vi "stop.vi"(8 "error in (no error)":errorcluster, 9 "InternalCommandId.lvclass":refnum<class "InternalCommandId.lvclass">, 10 "ElectrometerController in":refnum<class "ElectrometerController.lvclass">, 11 "UntilIntensityReading in":refnum<class "UntilIntensityReading.lvclass">) -> (0 "error out":errorcluster, 2 "ElectrometerController out":refnum<class "ElectrometerController.lvclass">, 3 "UntilIntensityReading out":refnum<class "UntilIntensityReading.lvclass">)   [LabVIEW 2016, in "UntilIntensityReading.lvclass"]
uses:
  UntilIntensityReading.lvclass
  ElectrometerController/ElectrometerController.lvclass
  InternalCommandId/InternalCommandId.lvclass
  ts_electrometeruserevents/Typedefs/StateValue.ctl
  ElectrometerController/ElectrometerController.lvclass/ElectrometerController.ctl
  ElectrometerState.lvclass
  ts_electrometeruserevents/Typedefs/ElectrometerTypedefs.lvlib
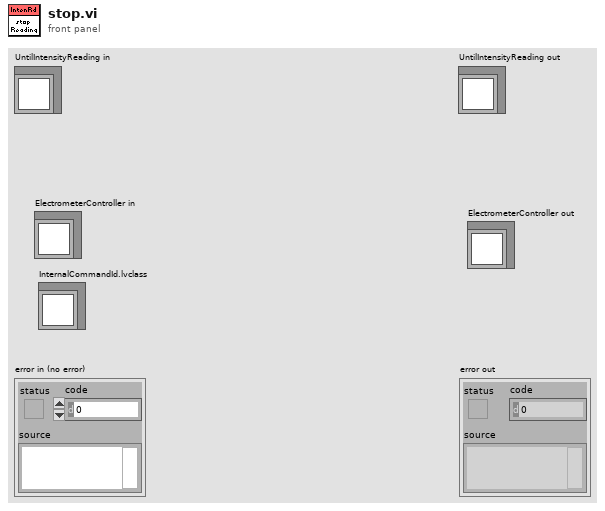
[diagram p1: front panel]
types:
  T1 = typedef "ElectrometerTypedefs.lvlib/StateValue.ctl" = enum16{"", "DisabledState", "EnabledState", "FaultState", "OffState", "StandbyState", "ReadyState", "ConfiguringState", "ManualReadingState", "UntilIntensityReadingState", "SetDurationReadingState", "BufferReadingState"}
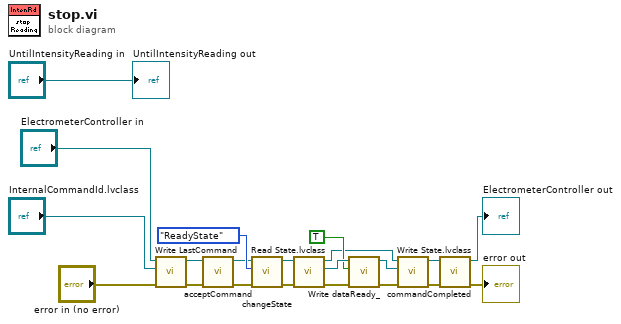
[diagram p0: block diagram]
diagram:
  n1 = call "Write LastCommand.vi"("error in (no error)"="error in (no error)", "InternalCommandId.lvclass"="InternalCommandId.lvclass", "ElectrometerController in"="ElectrometerController in") -> ("error out"=w7:errorcluster, "ElectrometerController out"=w8:refnum<class "ElectrometerController.lvclass">)  [unwired: 7 in]
  n2 = call "acceptCommand.vi"("error in (no error)"=w7, "ElectrometerController in"=w8) -> ("error out"=w6:errorcluster, "ElectrometerController out"=w5:refnum<class "ElectrometerController.lvclass">)  [unwired: 8 in]
  n3 = call "changeState.vi"("error in (no error)"=w6, "StateValue"=StateValue."ReadyState", "ElectrometerController in"=w5) -> ("error out"=w19:errorcluster, "ElectrometerController out"=w20:refnum<class "ElectrometerController.lvclass">)  [unwired: 7 in]
  n4 = call-dynamic "Read State.lvclass.vi"("error in (no error)"=w19, "ElectrometerController in"=w20) -> ("error out"=w17:errorcluster, "ElectrometerState"=w18:refnum<class "ElectrometerState.lvclass">, "ElectrometerController out"=w14:refnum<class "ElectrometerController.lvclass">)  [unwired: 7 in]
  n5 = call-dynamic "Write dataReady_.vi"("error in (no error)"=w17, "dataReady?"=TRUE, "State in"=w18) -> ("error out"=w13:errorcluster, "State out"=w15:refnum<class "ElectrometerState.lvclass">)  [unwired: 7 in]
  n6 = call-dynamic "Write State.lvclass.vi"("error in (no error)"=w13, "ElectrometerState"=w15, "ElectrometerController in"=w14) -> ("error out"=w3:errorcluster, "ElectrometerController out"=w4:refnum<class "ElectrometerController.lvclass">)  [unwired: 7 in]
  n7 = call "commandCompleted.vi"("error in (no error)"=w3, "ElectrometerController in"=w4) -> ("error out"=→"error out":errorcluster, "ElectrometerController out"=→"ElectrometerController out":refnum<class "ElectrometerController.lvclass">)  [unwired: 8 in]
  "UntilIntensityReading out" <- "UntilIntensityReading in"
